vi "bigcryo_single_RT.vi"(0 "Lake shore":refnum<visa-resource-name>="COM7", 5 "Keithley":refnum<visa-resource-name>="GPIB1::20::INSTR", 7 "File name":string="C:\\User Data\\hlb54\\NTS004\\NTS004_Tc_set=0.60T_9.txt", 9 "Set Sample Temp [K]":dbl=5.0, 11 "Reset":bool, 12 "Rate  [K/min]":dbl=0.25) -> (4 "R-H":cluster{"X":dbl[], "Y":dbl[]}[](graph) caption="XY Graph", 6 "Sample Temp [K]":dbl=5.0095, 8 "R":dbl=4.88350015e-05)   [LabVIEW 2019]
uses:
  <vilib>/express/express shared/transition.llb/Dynamic To Waveform Array.vi
  <vilib>/express/express signal manip/GetorSetDDTAttributes/Set DDT Attributes/SetT0.vi
  <vilib>/express/express shared/transition.llb/Waveform Array To Dynamic.vi
  <vilib>/express/express signal manip/GetorSetDDTAttributes/Set DDT Attributes/Set DDT Properties.xnode
panel:
  in  "Tol":dbl=0.2
  out "XY Graph":cluster{"X":dbl[], "Y":dbl[]}[](graph)
  out "VTI Temp [K]":dbl=5.0095
  out "Magnet Field":dbl=5.0095
  in  "Magnet":refnum<visa-resource-name>="COM6"
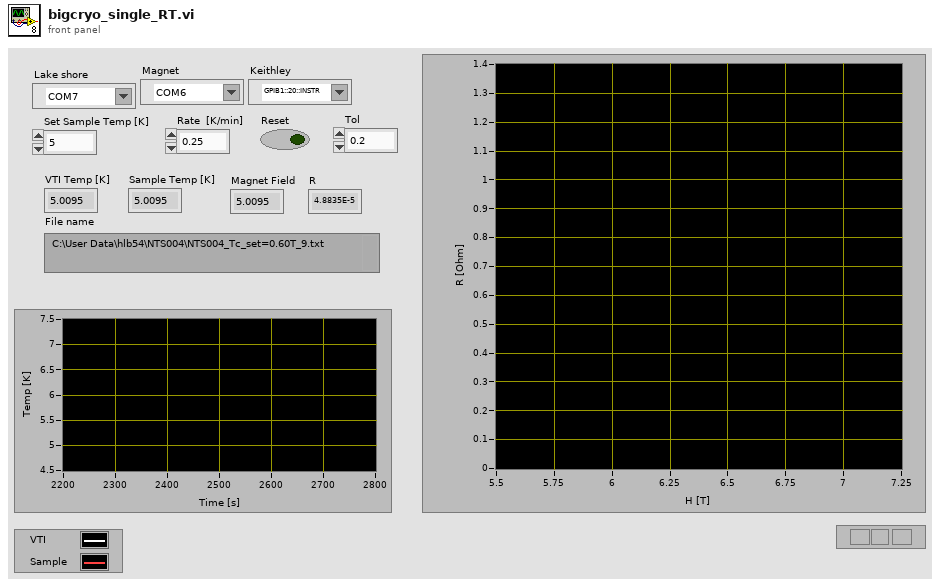
[diagram p1: front panel]
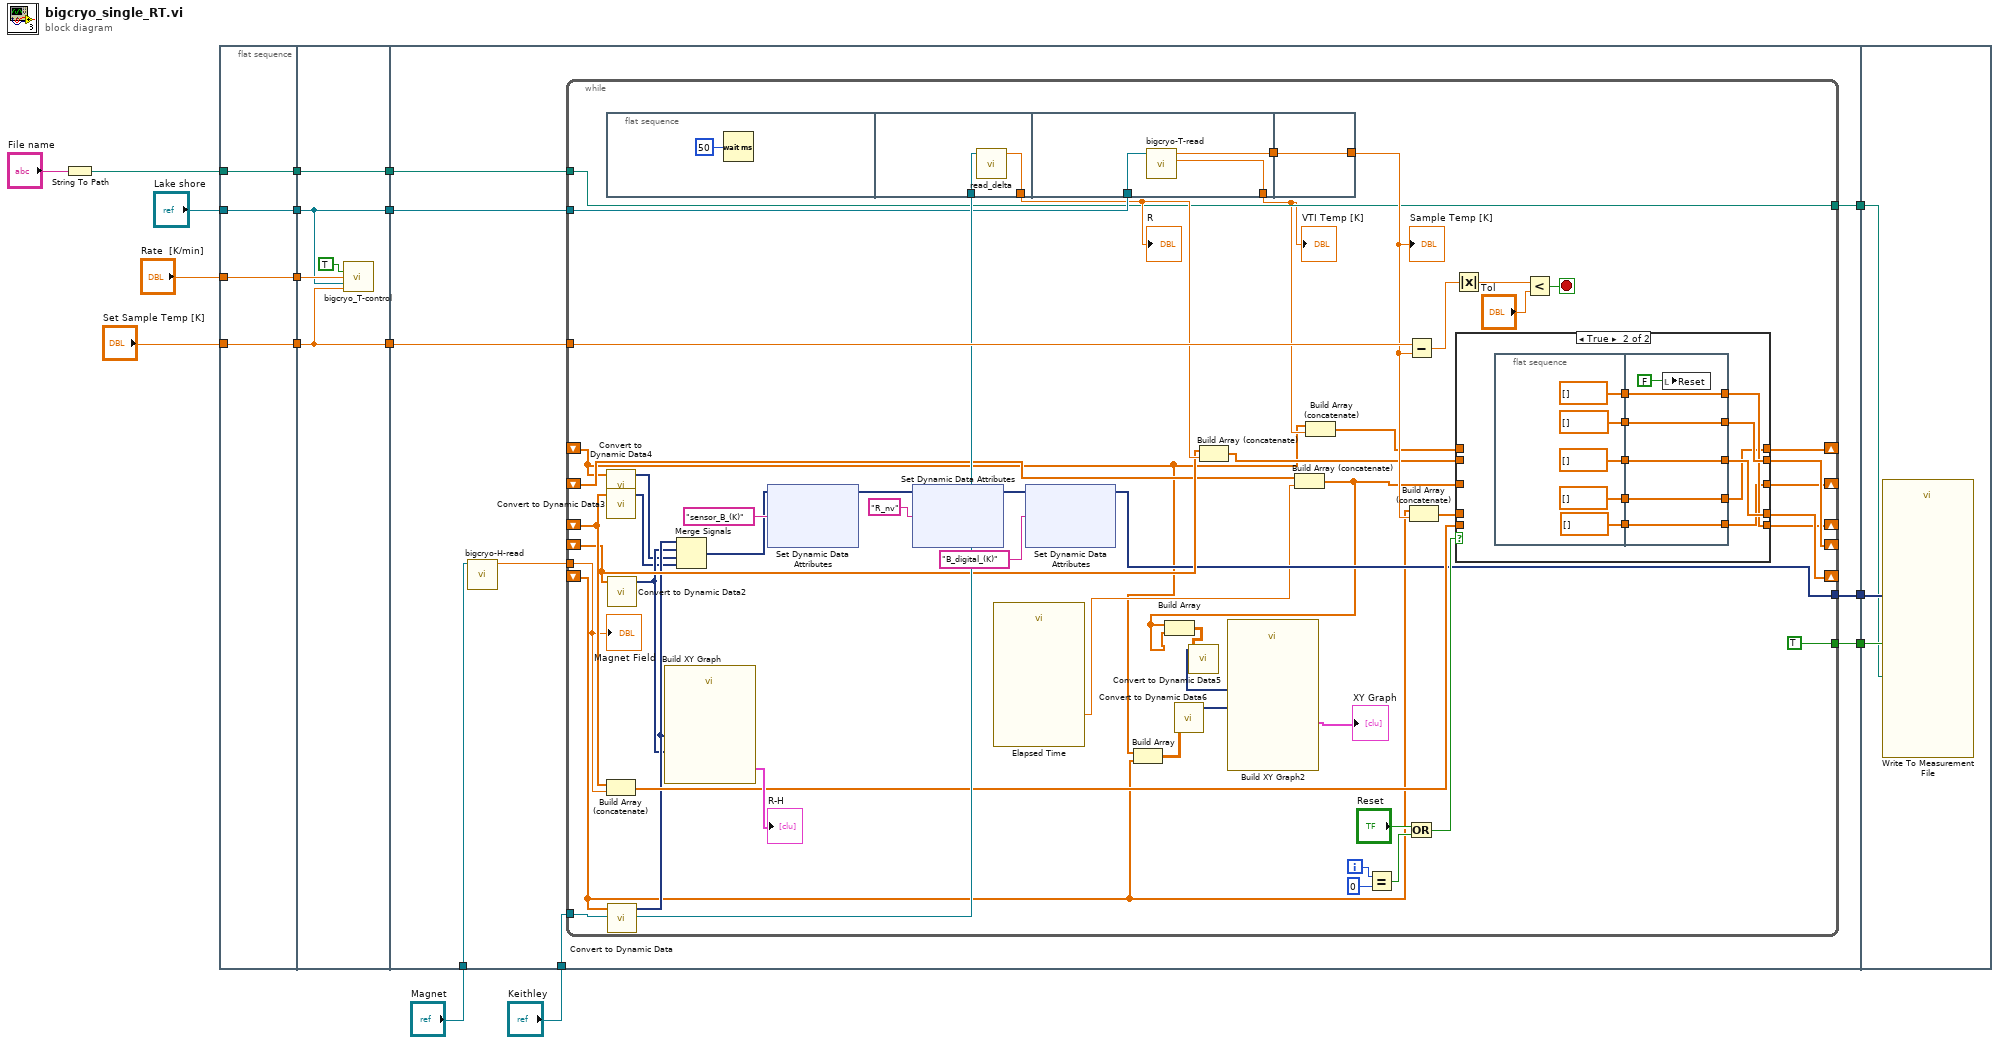
[diagram p0: block diagram]
diagram:
  n1 = String To Path(string="File name") -> (path=w14:path)
  n2 = flat-sequence {
    tunnel: "Lake shore" -> [w18]
    tunnel: "Rate  [K/min]" -> [w19]
    tunnel: w14 -> [w20]
    tunnel: "Set Sample Temp [K]" -> [w21]
    tunnel: [w21] -> w9
    tunnel: [w20] -> w8
    tunnel: [w19] -> w7
    tunnel: [w18] -> w6
    tunnel: [w26] -> w16
    tunnel: [w25] -> w15
    tunnel: [w22] -> w10
    tunnel: w9 -> [w26]
    tunnel: w8 -> [w25]
    tunnel: w7 -> [w24]
    tunnel: w6 -> [w22]
    tunnel: w16 -> [w35]
    tunnel: w15 -> [w34]
    tunnel: "Keithley" -> [w33]
    tunnel: w10 -> [w32]
    tunnel: [w31] -> w4
    tunnel: [w30] -> w3
    tunnel: [w29] -> w2
    tunnel: "Magnet" -> [w27]
    tunnel: w4 -> [w165]
    tunnel: w3 -> [w164]
    tunnel: w2 -> [w163]
    frame #0 {
    }
    frame #1 {
      n3 = call "bigcryo_T-control.vi"("Ramp Mode"=TRUE, "Rate  [K/min]"=w24, "VISA resource name out"=w22, "Set Sample Temp [K]"=w26) -> ()  [unwired: 12 in]
    }
    frame #2 {
      n4 = call "bigcryo-H-read.vi"("Magnet Power supply"=w27) -> ("Magnetic Field [T]"=w28:dbl)  [unwired: 10 in]
      n5 = while {
        shift-right: [w79] -> _
        shift-left: _ -> [w41]
        shift-right: [w78] -> _
        shift-left: _ -> [w63]
        tunnel: w35 -> [w87]
        tunnel: w34 -> [w70]
        tunnel: w33 -> [w82]
        tunnel: w32 -> [w81]
        tunnel: [w55] -> w31
        tunnel: [TRUE ("Enable")] -> w30
        tunnel: [w70] -> w29
        shift-right: [w67] -> _
        shift-left: _ -> [w66]
        tunnel: w28 -> [w65]
        shift-right: [w52] -> _
        shift-left: _ -> [w40]
        shift-right: [w45] -> _
        shift-left: _ -> [w44]
        i -> [w74]
        stop <- w84 stop-if-true
        n6 = flat-sequence {
          tunnel: [w158] -> w77
          tunnel: w82 -> [w157]
          tunnel: w81 -> [w160]
          tunnel: [w161] -> w69
          tunnel: [w159] -> w51
          tunnel: [w162] -> w80
          tunnel: w69 -> [w162]
          frame #0 {
            n7 = Wait (ms)(milliseconds to wait=50) -> ()  [unwired: 1 out]
          }
          frame #1 {
            n8 = call "read_delta.vi"("Keithley"=w157) -> ("delta reading [ohm]"=w158:dbl)  [unwired: 9 in, 1 out]
          }
          frame #2 {
            n9 = call "bigcryo-T-read.vi"("VISA resource name out"=w160) -> ("VTI Temp [K]"=w159:dbl, "Sample Temp [K]"=w161:dbl)  [unwired: 9 in]
          }
          frame #3 {
          }
        }
        n10 = call "Convert to Dynamic Data4"("Array"=w40) -> ("Dynamic Data Type"=w49:dynamicdata)  [unwired: 3 in]
        n11 = call "Convert to Dynamic Data3"("Array"=w66) -> ("Dynamic Data Type"=w53:dynamicdata)  [unwired: 3 in]
        n12 = Build Array (concatenate)(w66, w65) -> (w68:dbl[])
        n13 = call "Convert to Dynamic Data2"("Array"=w63) -> ("Dynamic Data Type"=w54:dynamicdata)  [unwired: 3 in]
        n14 = call "Convert to Dynamic Data"("Array"=w41) -> ("Dynamic Data Type"=w59:dynamicdata)  [unwired: 3 in]
        n15 = call "Build XY Graph"("Y Input"=w54, "X Input"=w59) -> ("XY Graph"=→"R-H":cluster{"X":dbl[], "Y":dbl[]}[])  [unwired: 8 in, 1 out]
        n16 = Merge Signals(w59, w54, w49, w53) -> (w58:dynamicdata)
        n17 = xnode "Set Dynamic Data Attributes"("Signals In"=w58, "Signal Name"="sensor_B_(K)") -> ("Signals Out"=w57:dynamicdata)  [unwired: 2 in, 1 out]
        n18 = xnode "Set Dynamic Data Attributes"("Signals In"=w57, "Signal Name"="R_nv") -> ("Signals Out"=w56:dynamicdata)  [unwired: 2 in, 1 out]
        n19 = call "Elapsed Time"() -> ("Elapsed Time (s)"=w43:dbl)  [unwired: 12 in, 7 out]
        n20 = xnode "Set Dynamic Data Attributes"("Signals In"=w56, "Signal Name"="B_digital_(K)") -> ("Signals Out"=w55:dynamicdata)  [unwired: 2 in, 1 out]
        n21 = Build Array(w40, w41) -> (w39:dbl[][])
        n22 = call "Convert to Dynamic Data6"("2D Array"=w39) -> ("Dynamic Data Type"=w47:dynamicdata)  [unwired: 3 in]
        n23 = Build Array (concatenate)(w63, w77) -> (w64:dbl[])
        n24 = Build Array (concatenate)(w44, w43) -> (w38:dbl[])
        n25 = Build Array(w38, w38) -> (w37:dbl[][])
        n26 = call "Convert to Dynamic Data5"("2D Array"=w37) -> ("Dynamic Data Type"=w46:dynamicdata)  [unwired: 3 in]
        n27 = call "Build XY Graph2"("Y Input"=w47, "X Input"=w46) -> ("XY Graph"=→"XY Graph":cluster{"X":dbl[], "Y":dbl[]}[])  [unwired: 8 in, 1 out]
        n28 = Build Array (concatenate)(w40, w51) -> (w50:dbl[])
        n29 = Equal?(x=w74, y=0) -> (x = y?=w72:bool)
        n30 = Subtract(x=w87, y=w80) -> (x-y=w86:dbl)
        n31 = Or(x="Reset", y=w72) -> (x .or. y?=w76:bool)
        n32 = Build Array (concatenate)(w41, w80) -> (w42:dbl[])
        n33 = Absolute Value(x=w86) -> (abs(x)=w85:dbl)
        n34 = case shown="True" w76 {
          tunnel: w64 -> [w134 _]
          tunnel: [w133 w144] -> w79
          tunnel: [w134 w143] -> w78
          tunnel: w42 -> [w133 _]
          tunnel: w68 -> [w132 _]
          tunnel: [w132 w139] -> w67
          tunnel: [w131 w137] -> w52
          tunnel: w50 -> [w131 _]
          tunnel: w38 -> [w130 _]
          tunnel: [w130 w135] -> w45
          frame False {
          }
          frame True {
            n35 = flat-sequence {
              tunnel: [dbl[] []] -> w142
              tunnel: [dbl[] []] -> w141
              tunnel: [dbl[] []] -> w140
              tunnel: [dbl[] []] -> w138
              tunnel: [dbl[] []] -> w136
              tunnel: [w154] -> w143
              tunnel: [w155] -> w144
              tunnel: w142 -> [w155]
              tunnel: w141 -> [w154]
              tunnel: w140 -> [w152]
              tunnel: [w152] -> w139
              tunnel: [w151] -> w137
              tunnel: w138 -> [w151]
              tunnel: w136 -> [w150]
              tunnel: [w150] -> w135
              frame #0 {
              }
              frame #1 {
                n36 = local write "Reset"(FALSE) -> ()
              }
            }
          }
        }
        n37 = Less?(x=w85, y="Tol") -> (x < y?=w84:bool)
        "Sample Temp [K]" <- w80
        "R" <- w77
        "Magnet Field" <- w65
        "VTI Temp [K]" <- w51
      }
    }
    frame #3 {
      n38 = call "Write To Measurement File"("Signals"=w165, "Enable"=w164, "Filename"=w163) -> ()  [unwired: 14 in, 3 out]
    }
  }
